vi "Comet Page.vi"() -> ()   [LabVIEW 2017, in "3D Comet.lvclass"]
uses:
  <vilib>/Math Plots/3D Math Plots/3D Comet/3D Comet/3D Comet.lvclass
  <vilib>/Math Plots/3D Math Plots/3D Comet/3D Comet/Typedef/3D Comet Property Array.ctl
  <vilib>/Math Plots/3D Math Plots/3D Comet/3D Comet/Typedef/3D Comet Property.ctl
  <vilib>/Math Plots/3D Math Plots/3D Plot/3D Plot/Typedef/Sprite Type.ctl
  <vilib>/Math Plots/3D Math Plots/3D Plot/3D Plot/Typedef/Line Type.ctl
  <vilib>/Math Plots/3D Math Plots/3D Plot/3D Plot/Typedef/Dialog State.ctl
  <vilib>/Math Plots/3D Math Plots/3D Plot/3D Plot/Typedef/Temp Scene State.ctl
  <vilib>/Math Plots/3D Math Plots/3D Plot/3D Plot/Typedef/Temp Scene Property Action.ctl
  <vilib>/Math Plots/3D Math Plots/3D Plot/3D Plot/3D Plot.lvclass
panel:
  in  "Point Color":u32(colorbox) caption="Point color"
  in  "Point Size":sgl caption="Point size" min=0.001 step=1
  in  "Point Style":u16(ring) caption="Point style"
  in  "Tail Length":sgl caption="Tail length"
  in  "Line Style":u16(ring) caption="Line style"
  in  "Antialiasing":bool
  in  "Line Width":sgl=0.001 caption="Line width" min=0.001 step=1
  in  "Line Color":u32(colorbox) caption="Line color"
  out "Comet Property Out":T1
  in  "Comet Property In":T1
  in  "YZ Plane Projection":bool caption="YZ plane projection"
  in  "XZ Plane Projection":bool caption="XZ plane projection"
  in  "XY plane projection":bool
  in  "Coordinate System":u16(ring) caption="Coordinate system" items=["Cartesian", "Cylindrical", "Spherical"]
  in  "Plot Opacity":sgl(slide) caption="Plot opacity(%)" min=0 max=100 scale=0.0..100.0
  in  "Plot List":i32(listbox)
  in  "Move Down":bool
  in  "Move Up":bool
  in  "Delete":bool
  in  "New":bool
  in  "Event Registration":refnum<event-registration>
  # "Comet"
  # "General"
  # "Projection"
  # "Comet Line"
  # "Comet Point"
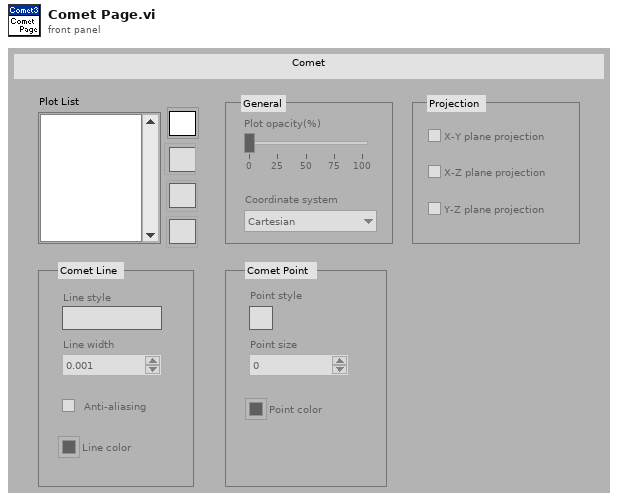
[diagram p1: front panel]
types:
  T1 = typedef "3D Comet.lvclass/3D Comet Property Array.ctl" = T2[]
  T2 = typedef "3D Comet.lvclass/3D Comet Property.ctl" = cluster{"General Property":cluster{"Plot Name":string, "Coordinate System":enum16{"Cartesian", "Cylindrical", "Spherical"}, "Opacity":sgl}, "Projection Property":cluster{"Draw XY":bool, "Draw YZ":bool, "Draw XZ":bool}, "Plot Property":cluster{"Sprite Type":T3, "Point Size":sgl, "Point Color":u32, "Line Style":T4, "Line Width":sgl, "Line Color":u32, "Antialiasing":bool}, "Comet Property":cluster{"Body length":sgl}}
  T3 = typedef "3D Plot.lvclass/Sprite Type.ctl" = enum16{"None", "Empty Square", "Solid Square", "Empty Diamond", "Solid Diamond", "Empty Circle", "Solid Circle", "Asterisk", "Bold X", "Wireframe Sphere", "Solid Sphere", "Wireframe Cube", "Solid Cube"}
  T4 = typedef "3D Plot.lvclass/Line Type.ctl" = enum16{"None", "Solid", "Dash", "Dot", "Dash Dot"}
  T5 = typedef "3D Plot.lvclass/Dialog State.ctl" = enum16{"Initialize", "Read Porperty", "Write Property", "Idle", "Exit"}
  T6 = typedef "3D Plot.lvclass/Temp Scene State.ctl" = enum16{"Create", "Update Scene", "Get Plot Representation", "Destory"}
  T7 = typedef "3D Plot.lvclass/Temp Scene Property Action.ctl" = enum16{"Graph Property", "Light Property", "Axis Property", "Value Pair Property", "Format Property", "Cursor Property", "Plot Specific Property"}
  T8 = typedef "3D Plot.lvclass/Multiplot Representation.ctl" = cluster{"Plot Represention Array":T9[], "Max Range":T10}
  T9 = typedef "3D Plot.lvclass/Plot Representation.ctl" = cluster{"Plot ID":i32, "Plot Range":T10, "Mesh Data":T11, "Dimension":cluster{"X Dimension":i32, "Y Dimension":i32}, "Ramp Range":T10}
  T10 = typedef "3D Plot.lvclass/Range Clusters.ctl" = cluster{"X Range":cluster{"Max X":sgl, "Min X":sgl}, "Y Range":cluster{"Max Y":sgl, "Min Y":sgl}, "Z Range":cluster{"Max Z":sgl, "Min Z":sgl}}
  T11 = typedef "3D Plot.lvclass/Mesh Data.ctl" = cluster{"Index Array":u32[], "Vertex Array":cluster{"X":sgl, "Y":sgl, "Z":sgl}[], "Normal Array":cluster{"X":sgl, "Y":sgl, "Z":sgl}[], "Color Index Array":i32[]}
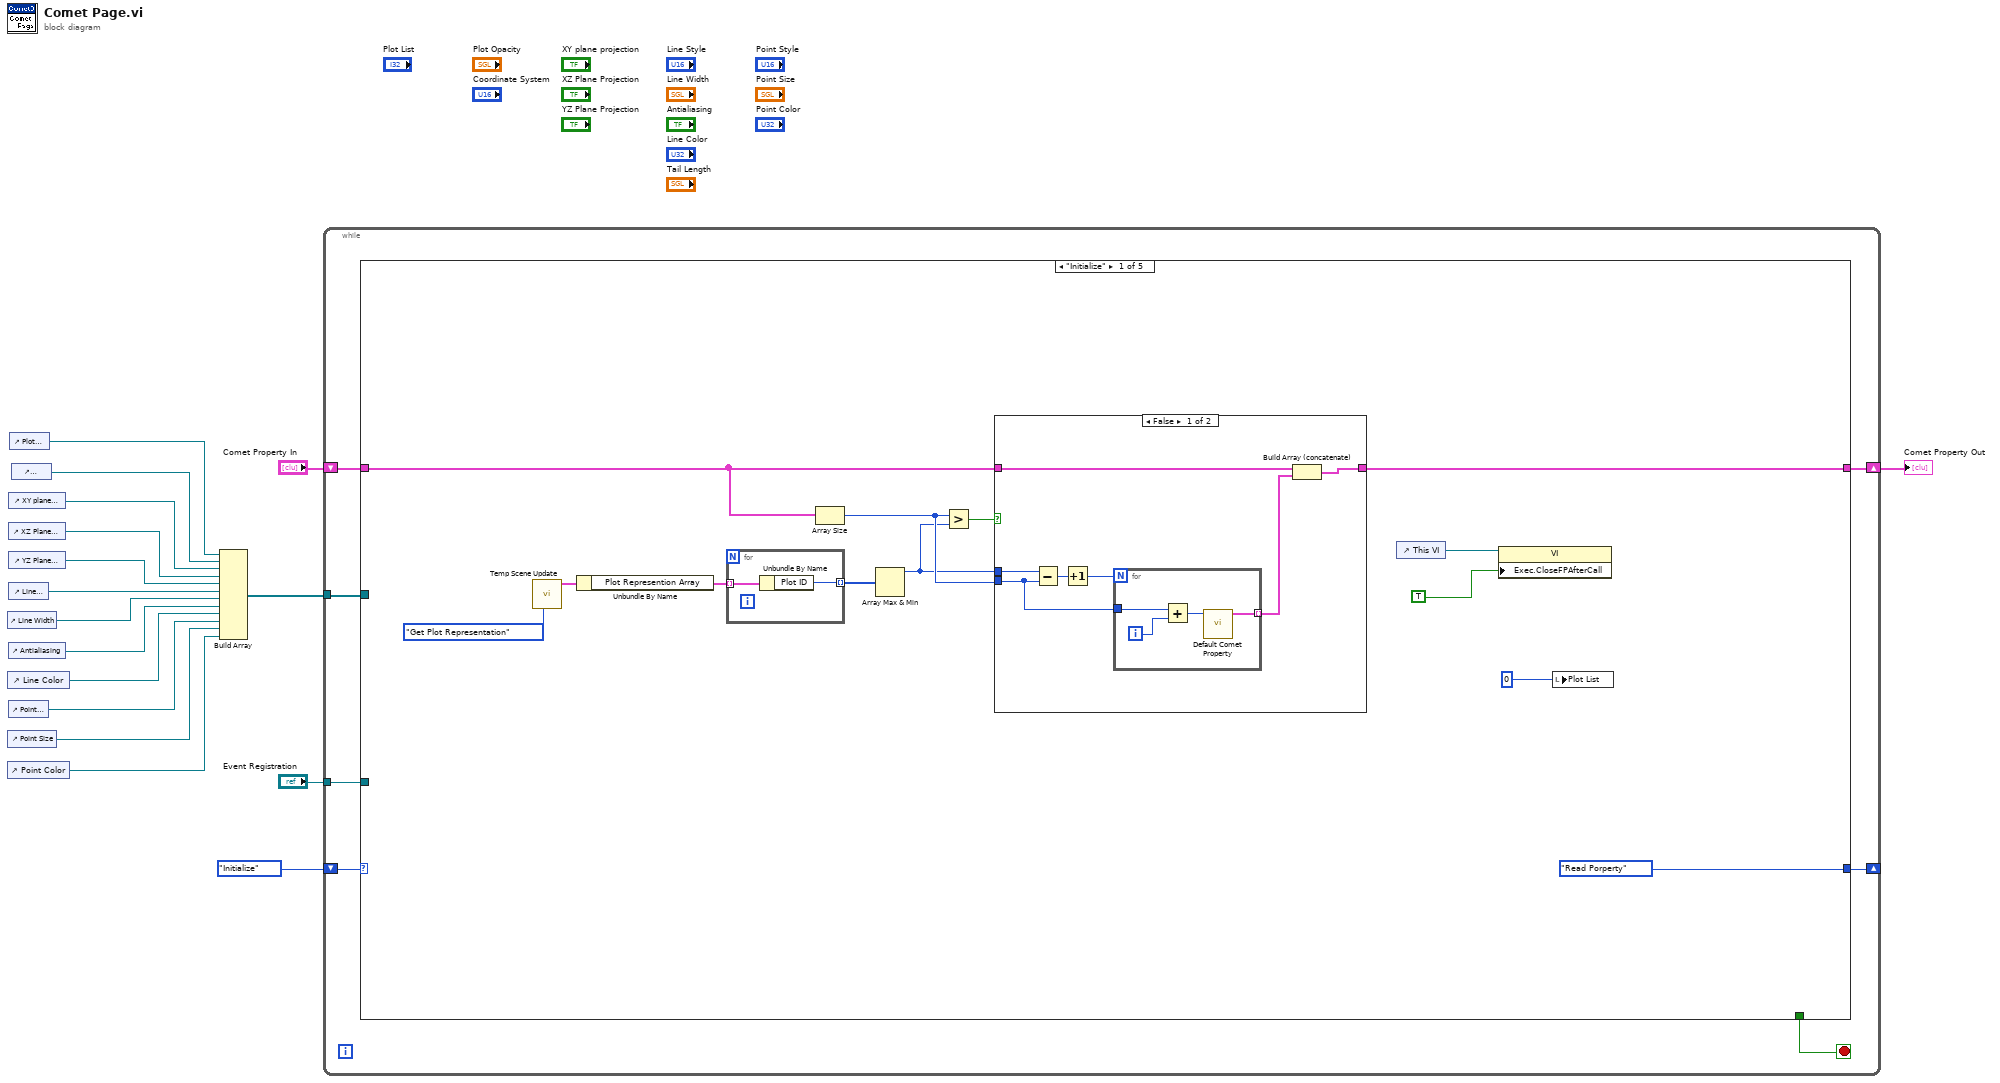
[diagram p0: block diagram]
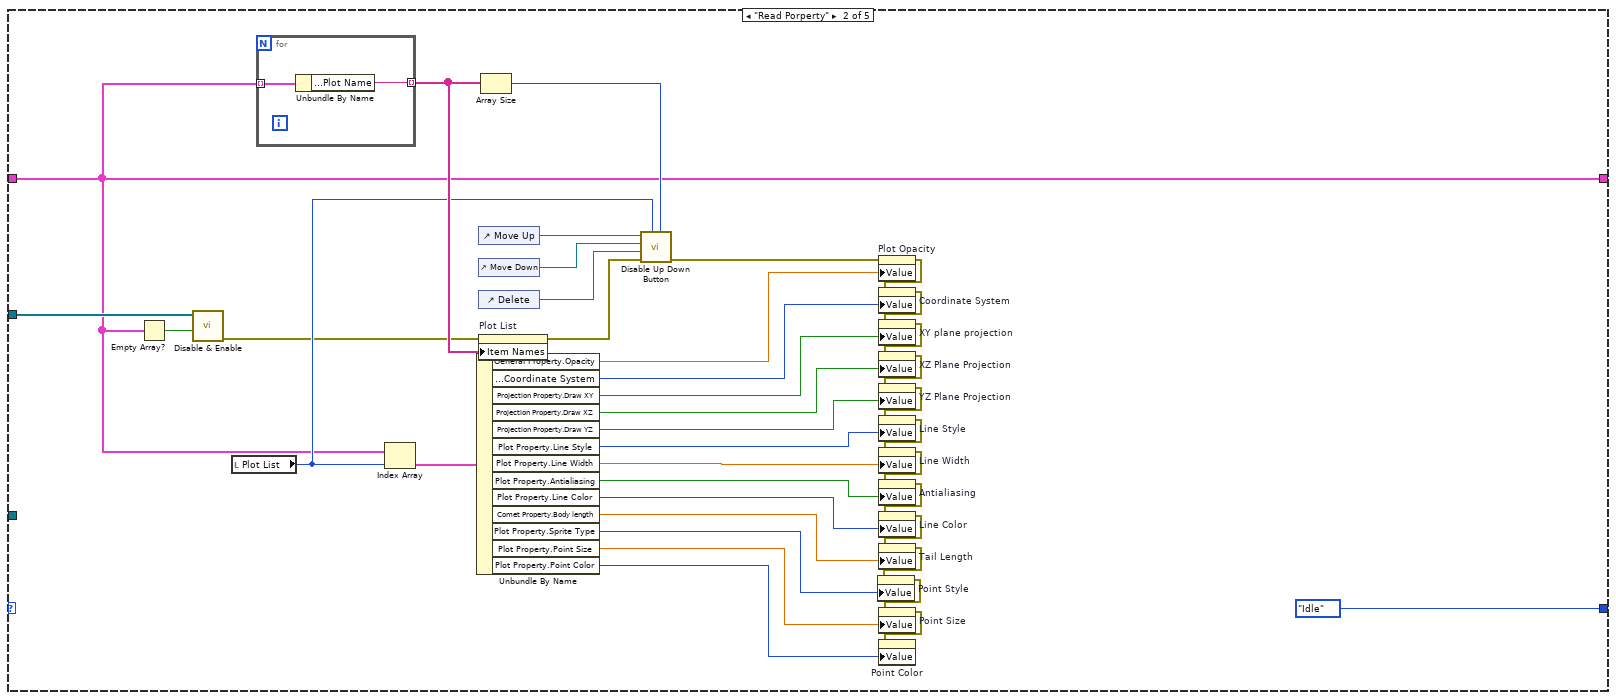
[diagram p3: hidden frame]
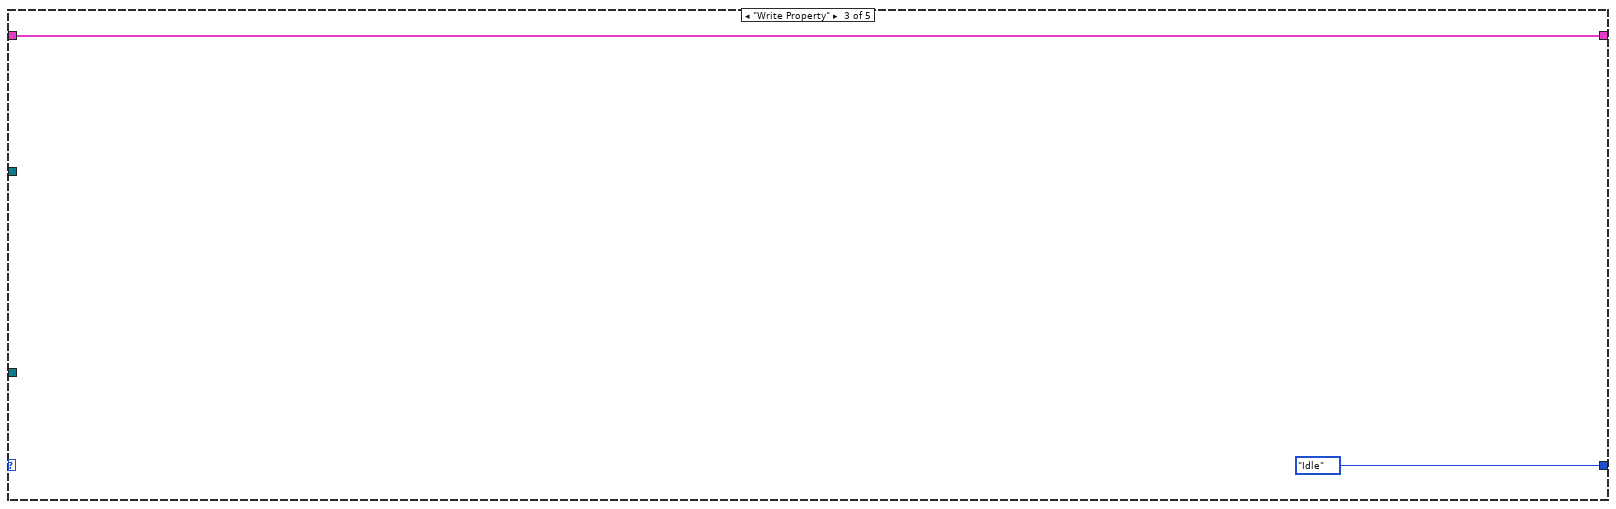
[diagram p4: hidden frame]
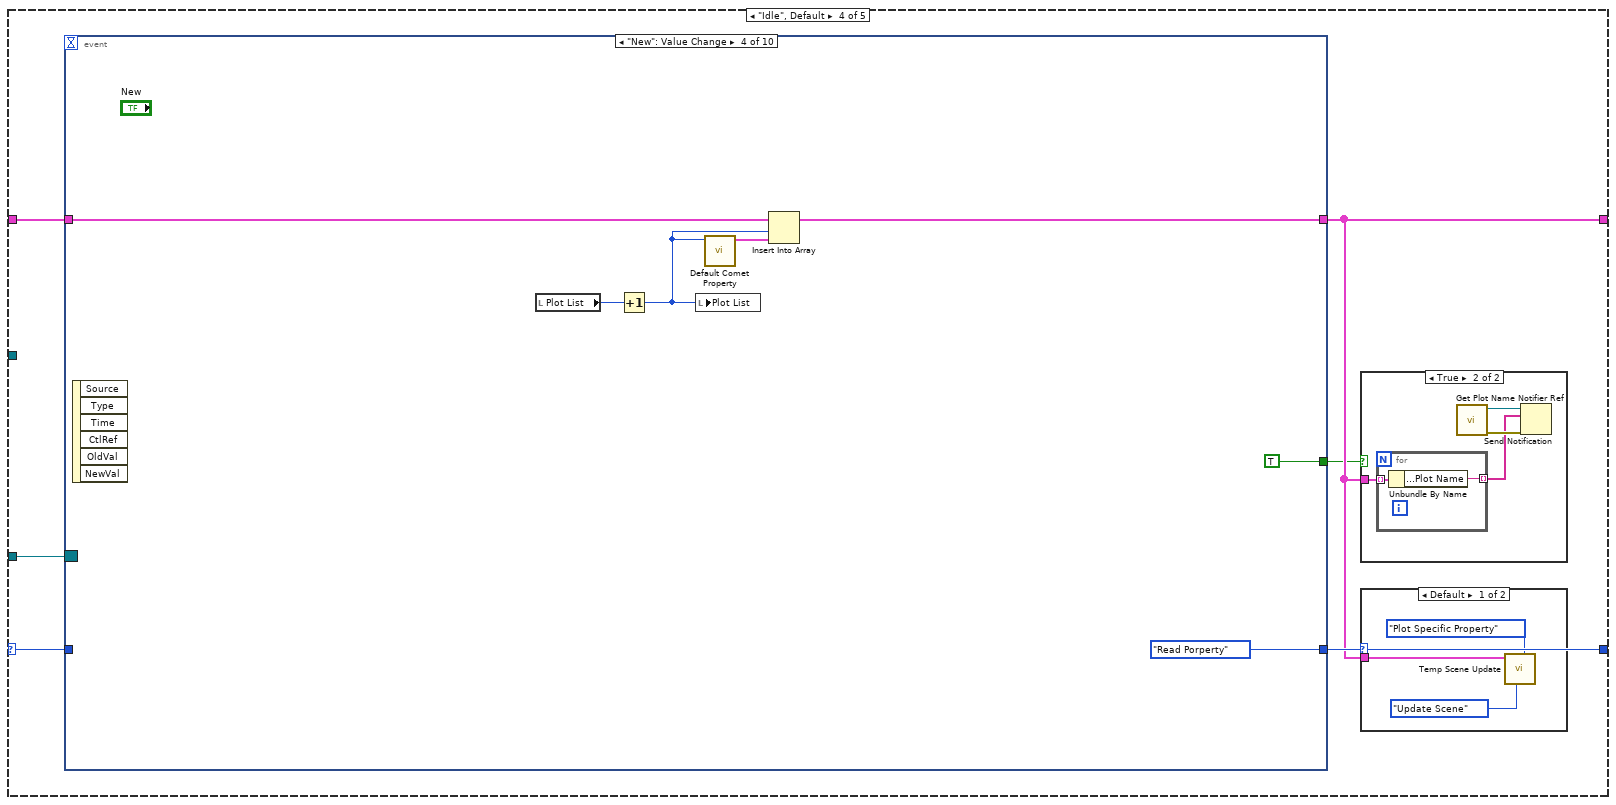
[diagram p5: hidden frame]
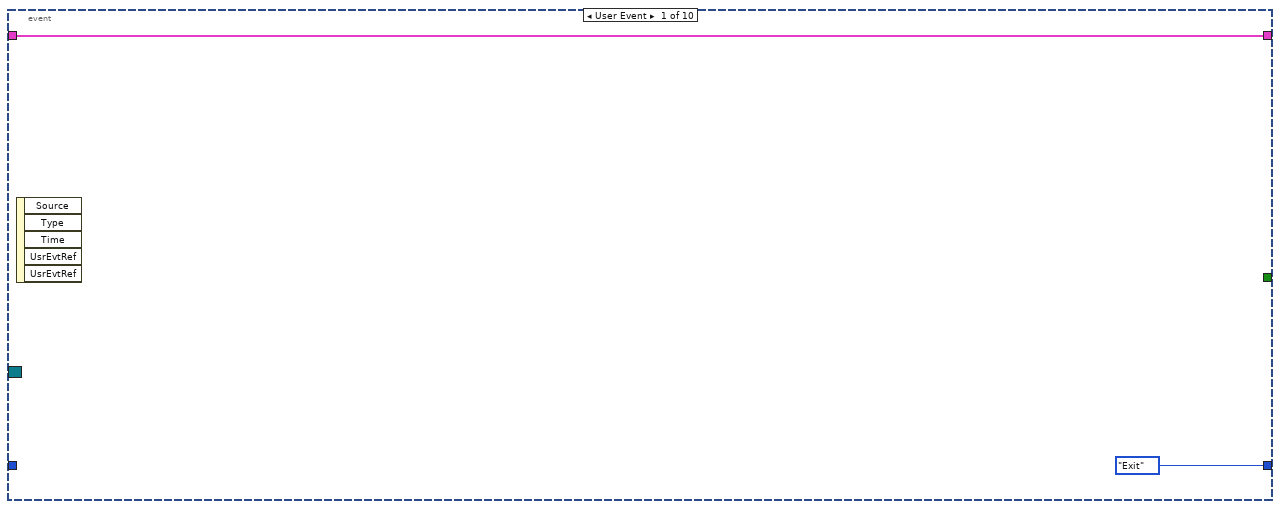
[diagram p8: hidden frame]
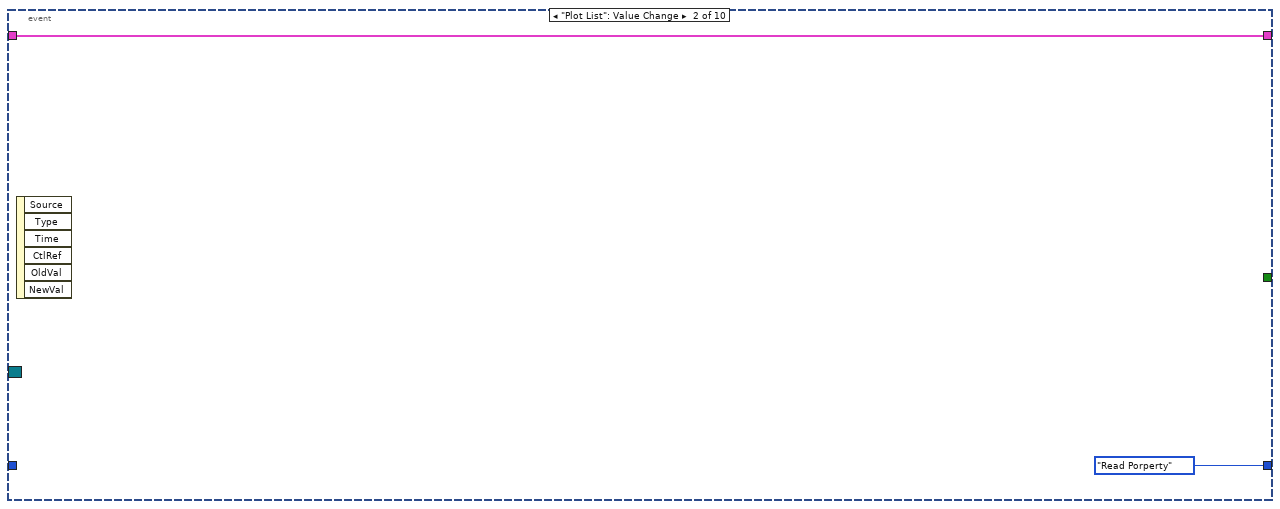
[diagram p9: hidden frame]
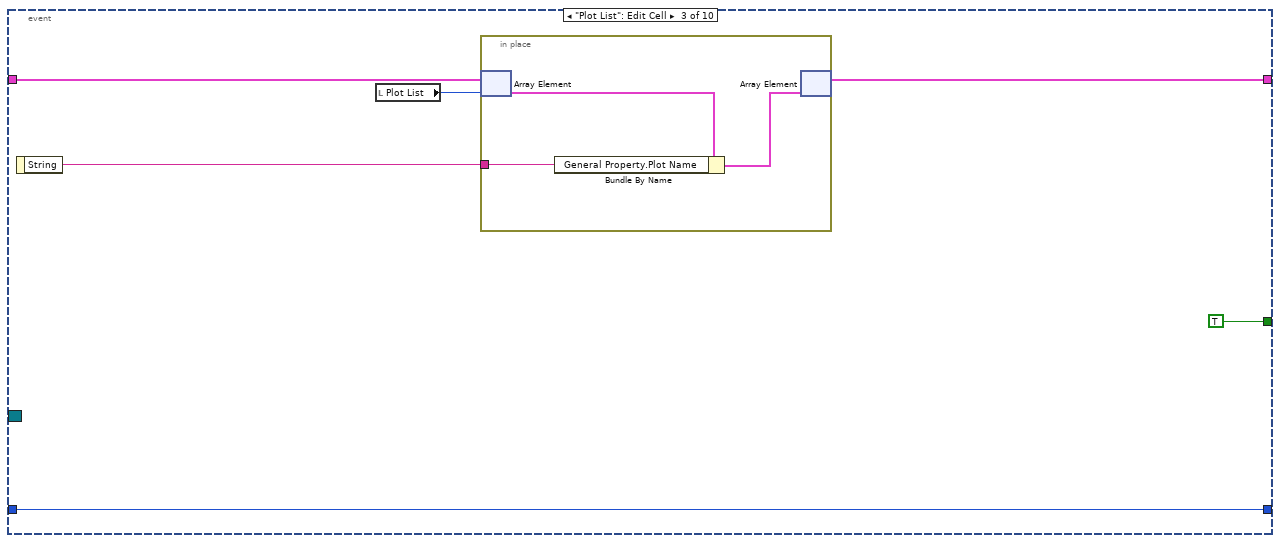
[diagram p10: hidden frame]
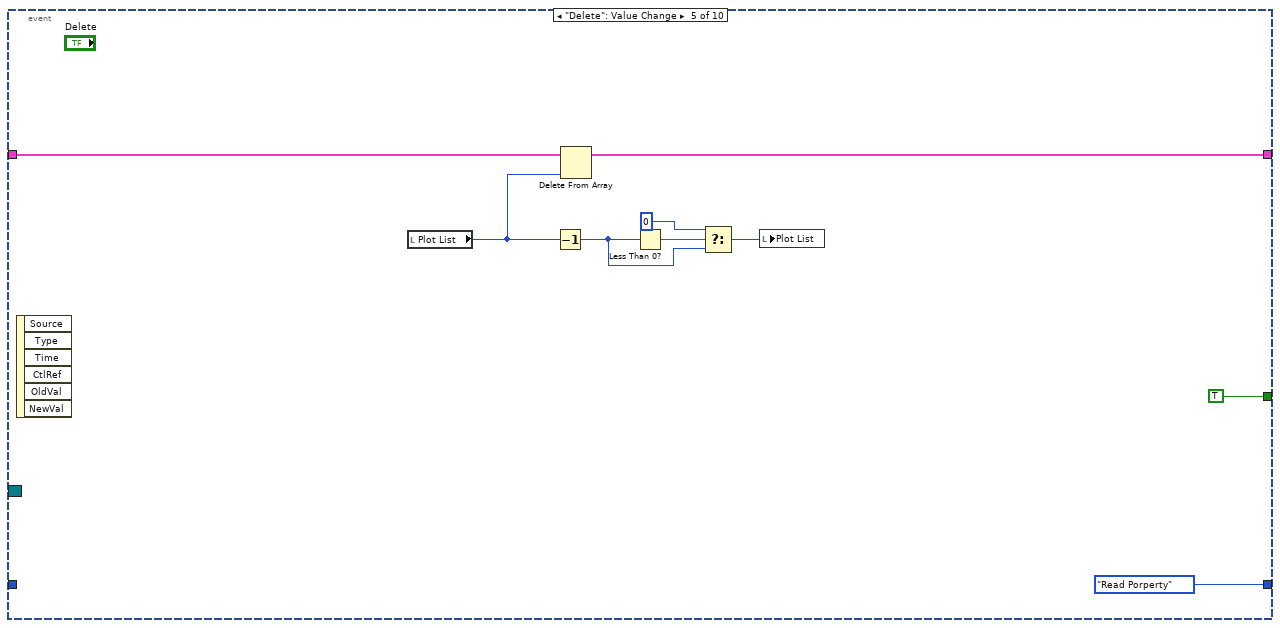
[diagram p11: hidden frame]
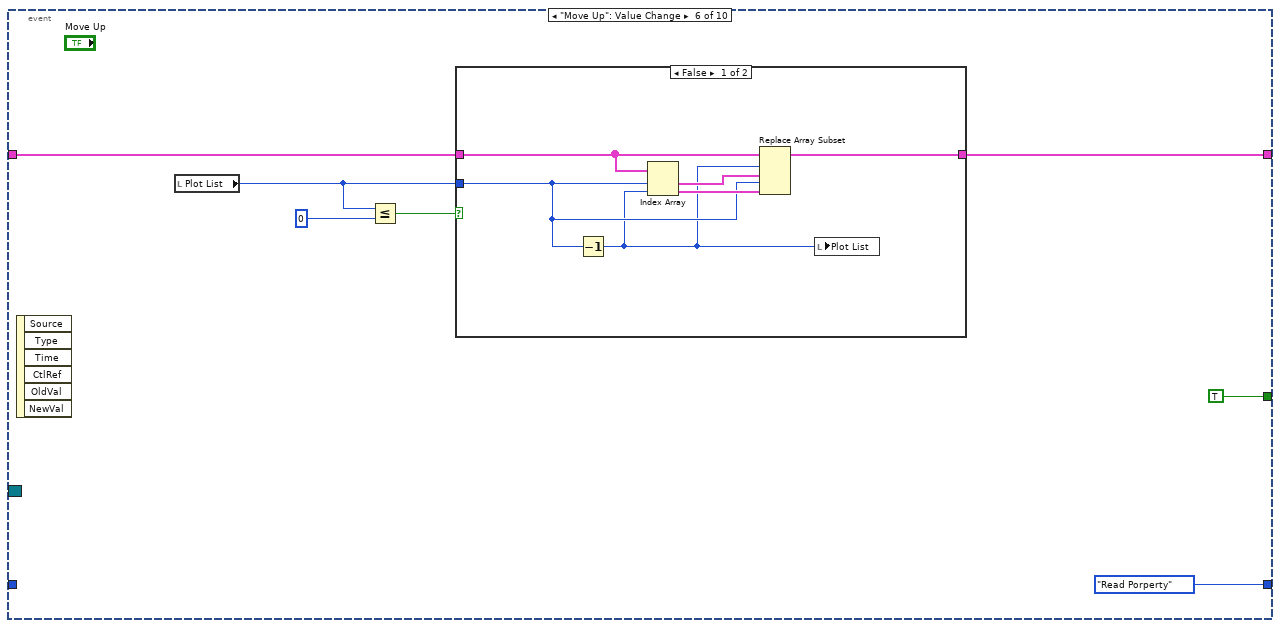
[diagram p12: hidden frame]
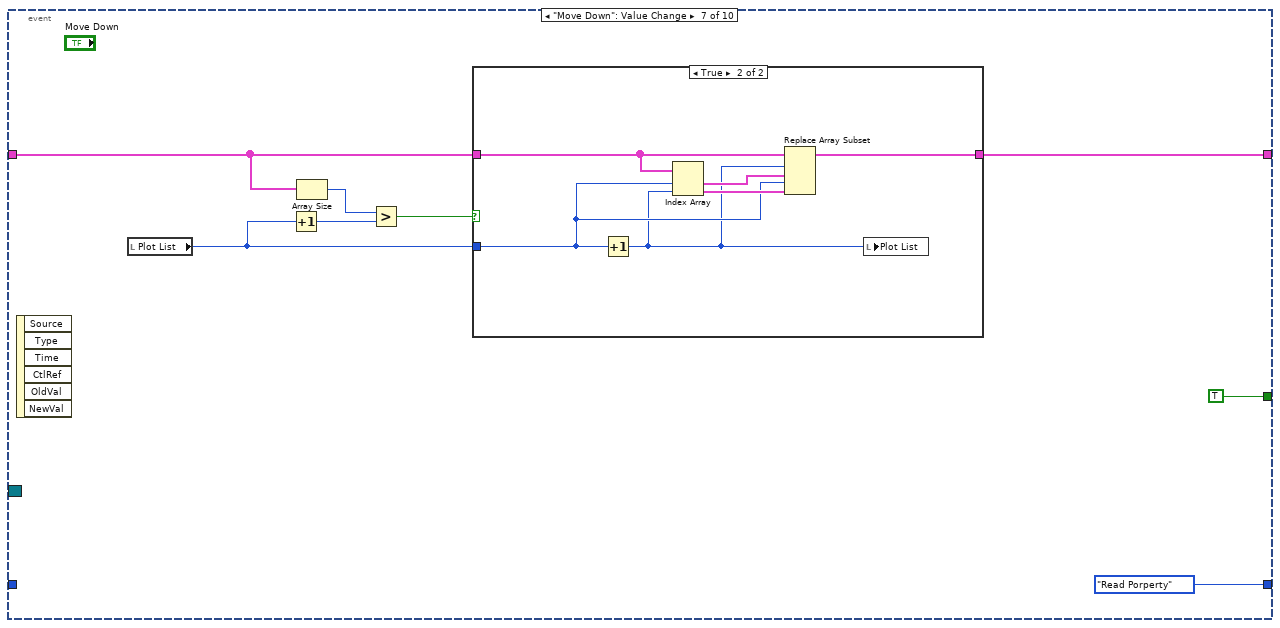
[diagram p14: hidden frame]
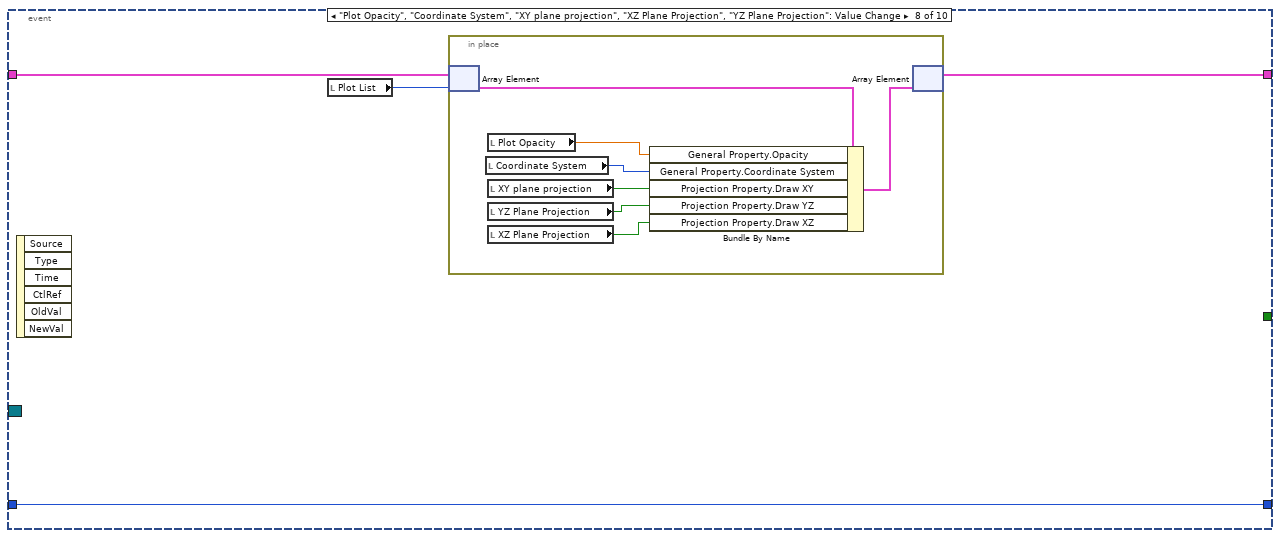
[diagram p16: hidden frame]
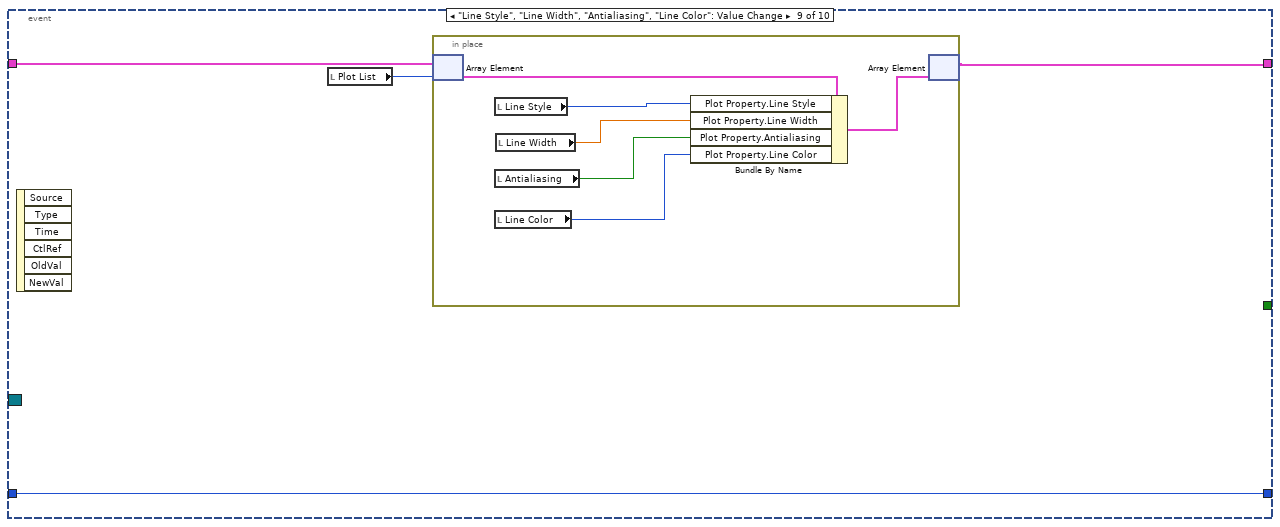
[diagram p17: hidden frame]
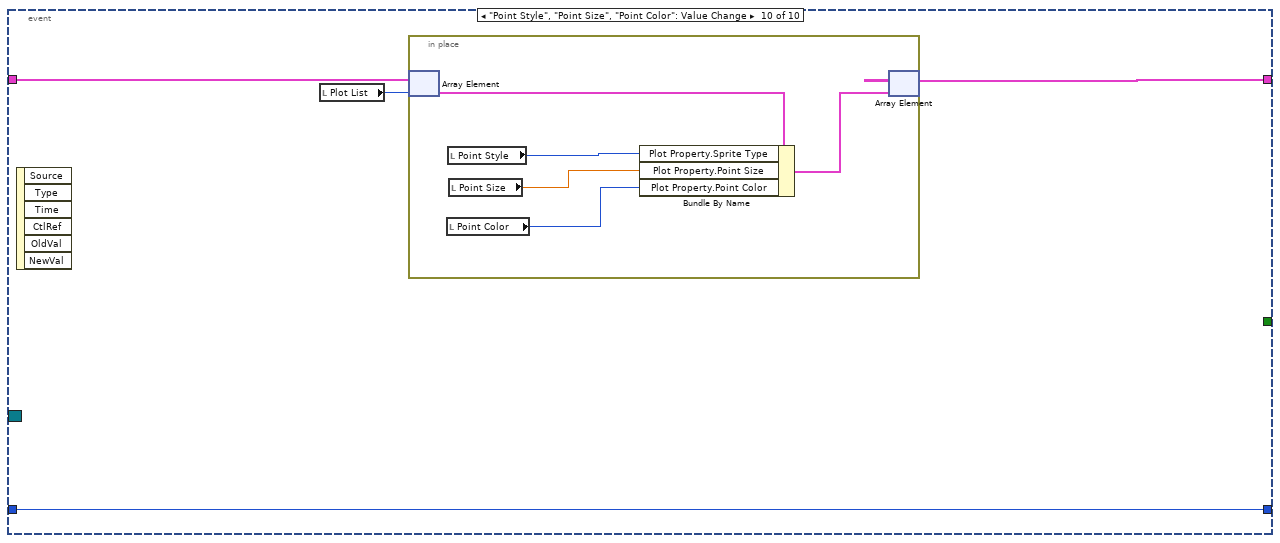
[diagram p18: hidden frame]
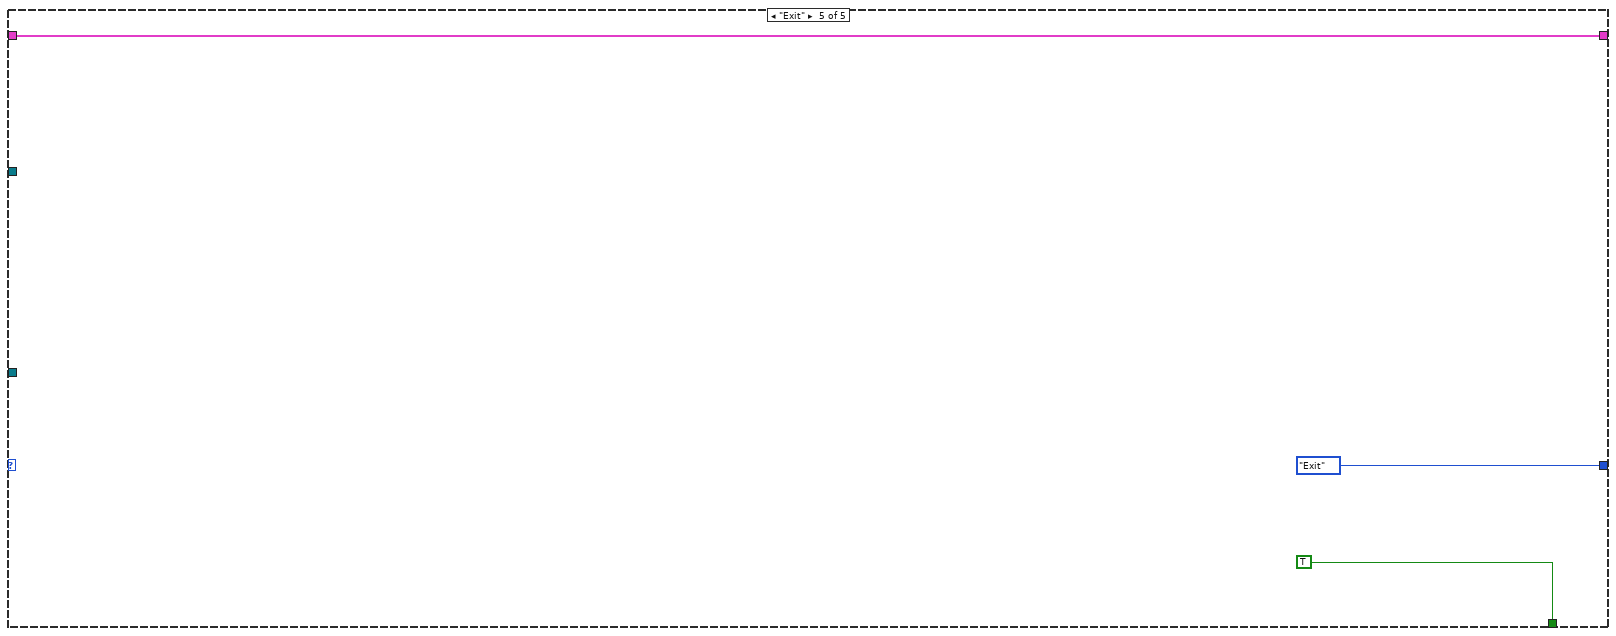
[diagram p19: hidden frame]
diagram:
  n1 = control-ref of="Line Width"() -> (w7:refnum<vi>)
  n2 = control-ref of="Line Color"() -> (w5:refnum<vi>)
  n3 = control-ref of="Point Size"() -> (w3:refnum<vi>)
  n4 = control-ref of="Point Color"() -> (w2:refnum<vi>)
  n5 = control-ref of="XY plane projection"() -> (w11:refnum<vi>)
  n6 = control-ref of="XZ Plane Projection"() -> (w10:refnum<vi>)
  n7 = control-ref of="YZ Plane Projection"() -> (w9:refnum<vi>)
  n8 = control-ref of="Line Style"() -> (w8:refnum<vi>)
  n9 = control-ref of="Antialiasing"() -> (w6:refnum<vi>)
  n10 = control-ref of="Point Style"() -> (w4:refnum<vi>)
  n11 = control-ref of="Plot Opacity"() -> (w13:refnum<vi>)
  n12 = control-ref of="Coordinate System"() -> (w12:refnum<vi>)
  n13 = Build Array(w13, w12, w11, w10, w9, w8, w7, w6, w5, w4, w3, w2) -> (w1:refnum<vi>[])
  n14 = while {
    shift-right: [w23] -> w14
    shift-left: "Comet Property In" -> [w24]
    shift-right: [w19] -> _
    shift-left: Dialog_State."Initialize" -> [w22]
    tunnel: "Event Registration" -> [w20]
    tunnel: w1 -> [w18]
    stop <- w21 stop-if-true
    n15 = case shown="\"Initialize\"" w22 {
      selector: w22 -> [_ _ _ w98 _]
      tunnel: w24 -> [w27 w79 w93 w100 w198]
      tunnel: [w26 w79 w93 w96 w198] -> w23
      tunnel: [Dialog_State."Read Porperty" Dialog_State."Idle" Dialog_State."Idle" w97 Dialog_State."Exit"] -> w19
      tunnel: [_ _ _ _ TRUE] -> w21
      tunnel: w20 -> [_ _ _ w99 _]
      tunnel: w18 -> [_ w80 _ _ _]
      frame "Initialize" {
        n16 = call <vilib>:"Temp Scene Update.vi"("State"=Temp_Scene_State."Get Plot Representation") -> ("Multiplot Representation"=w32:T8)  [unwired: 5 in, 5 out]
        n17 = Unbundle By Name(w32) -> ("Plot Represention Array"=w25:T9[])
        n18 = for {
          tunnel: w25 -> [w51] mode=indexing
          tunnel: [w50] -> w31 mode=indexing
          n19 = Unbundle By Name(w51) -> ("Plot ID"=w50:i32)
        }
        n20 = Array Size(array=w27) -> (size(s)=w29:i32)
        n21 = Array Max & Min(array=w31) -> (max value=w28:i32)  [unwired: 3 out]
        n22 = Greater?(x=w29, y=w28) -> (0:w30:bool)
        n23 = case shown="False" w30 {
          tunnel: [w42 w49] -> w26
          tunnel: w27 -> [w44 w49]
          tunnel: w29 -> [w38 _]
          tunnel: w28 -> [w39 _]
          frame False {
            n24 = Subtract(x=w39, y=w38) -> (x-y=w41:i32)
            n25 = Increment(x=w41) -> (x+1=w40:i32)
            n26 = for {
              N: w40 -> [_]
              tunnel: w38 -> [w47]
              tunnel: [w45] -> w43 mode=indexing
              i -> [w48]
              n27 = Add(x=w47, y=w48) -> (x+y=w46:i32)
              n28 = call <vilib>:"Default Comet Property.vi"("Plot ID"=w46) -> ("Default Property"=w45:T2)  [unwired: 10 out]
            }
            n29 = Build Array (concatenate)(w44, w43) -> (w42:T1)
          }
          frame True {
          }
        }
        n30 = control-ref of="This VI"() -> (w36:refnum<vi>)
        n31 = property class="VI"(reference=w36, "Exec.CloseFPAfterCall"=TRUE ("Execution:Close After Call")) -> ()  [unwired: 1 in, 2 out]
        n32 = local write "Plot List"(0 ("Plot List")) -> ()
      }
      frame "Read Porperty" {
        n33 = Empty Array?(array=w79) -> (empty?=w81:bool)
        n34 = call <vilib>:"Disable & Enable.vi"("Disabled?"=w81, "Control Ref Array"=w80) -> ("error out"=w78:errorcluster)  [unwired: 1 in, 8 out]
        n35 = local read "Plot List"() -> (w82:i32)
        n36 = for {
          tunnel: w79 -> [w92] mode=indexing
          tunnel: [w91] -> w84 mode=indexing
          n37 = Unbundle By Name(w92) -> ("General Property.Plot Name"=w91:string)
        }
        n38 = Index Array(array=w79, index=w82) -> (element=w89:T2)
        n39 = Unbundle By Name(w89) -> ("General Property.Opacity"=w67:sgl, "General Property.Coordinate System"=w66:enum16{"Cartesian", "Cylindrical", "Spherical"}, "Projection Property.Draw XY"=w65:bool, "Projection Property.Draw XZ"=w64:bool, "Projection Property.Draw YZ"=w63:bool, "Plot Property.Line Style"=w62:T4, "Plot Property.Line Width"=w61:sgl, "Plot Property.Antialiasing"=w60:bool, "Plot Property.Line Color"=w59:u32, "Comet Property.Body length"=w58:sgl, "Plot Property.Sprite Type"=w53:T3, "Plot Property.Point Size"=w57:sgl, "Plot Property.Point Color"=w56:u32)
        n40 = control-ref of="Move Up"() -> (w86:refnum<vi>)
        n41 = control-ref of="Move Down"() -> (w87:refnum<vi>)
        n42 = control-ref of="Delete"() -> (w88:refnum<vi>)
        n43 = property on="Plot List" class="LstBox (strict)"(error in=w78, "Item Names"=w84) -> (error out=w83:errorcluster)  [unwired: 1 in, 1 out]
        n44 = Array Size(array=w84) -> (size(s)=w85:i32)
        n45 = call <vilib>:"Disable Up Down Button.vi"("Length"=w85, "Index"=w82, "error in (no error)"=w83, "Delete Ref"=w88, "Move Down Ref"=w87, "Move Up Ref"=w86) -> ("error out"=w52:errorcluster)  [unwired: 5 out]
        n46 = property on="Plot Opacity" class="Slide (strict)"(error in=w52, "Value"=w67) -> (error out=w77:errorcluster)  [unwired: 1 in, 1 out]
        n47 = property on="Coordinate System" class="Ring (strict)"(error in=w77, "Value"=w66) -> (error out=w76:errorcluster)  [unwired: 1 in, 1 out]
        n48 = property on="XY plane projection" class="Bool (strict)"(error in=w76, "Value"=w65) -> (error out=w75:errorcluster)  [unwired: 1 in, 1 out]
        n49 = property on="XZ Plane Projection" class="Bool (strict)"(error in=w75, "Value"=w64) -> (error out=w74:errorcluster)  [unwired: 1 in, 1 out]
        n50 = property on="YZ Plane Projection" class="Bool (strict)"(error in=w74, "Value"=w63) -> (error out=w73:errorcluster)  [unwired: 1 in, 1 out]
        n51 = property on="Line Style" class="Ring (strict)"(error in=w73, "Value"=w62) -> (error out=w72:errorcluster)  [unwired: 1 in, 1 out]
        n52 = property on="Line Width" class="DigNum (strict)"(error in=w72, "Value"=w61) -> (error out=w71:errorcluster)  [unwired: 1 in, 1 out]
        n53 = property on="Antialiasing" class="Bool (strict)"(error in=w71, "Value"=w60) -> (error out=w70:errorcluster)  [unwired: 1 in, 1 out]
        n54 = property on="Line Color" class="ColBox"(error in=w70, "Value"=w59) -> (error out=w69:errorcluster)  [unwired: 1 in, 1 out]
        n55 = property on="Tail Length" class="DigNum (strict)"(error in=w69, "Value"=w58) -> (error out=w55:errorcluster)  [unwired: 1 in, 1 out]
        n56 = property on="Point Style" class="Ring (strict)"(error in=w55, "Value"=w53) -> (error out=w54:errorcluster)  [unwired: 1 in, 1 out]
        n57 = property on="Point Size" class="DigNum (strict)"(error in=w54, "Value"=w57) -> (error out=w68:errorcluster)  [unwired: 1 in, 1 out]
        n58 = property on="Point Color" class="ColBox"(error in=w68, "Value"=w56) -> ()  [unwired: 1 in, 2 out]
      }
      frame "Write Property" {
      }
      frame "Idle", Default {
        n59 = event shown="[3] \"New\": Value Change" {
          selector: w99 -> [_ _ _ _ _ _ _ _ _ _]
          dyn-events: _ -> [_ _ _ _ _ _ _ _ _ _]
          timeout: _ -> [_ _ _ _ _ _ _ _ _ _]
          tunnel: w100 -> [w111 w113 w117 w127 w136 w141 w155 w169 w180 w190]
          tunnel: [w111 w113 w116 w126 w137 w140 w154 w168 w179 w189] -> w96
          tunnel: [Dialog_State."Exit" Dialog_State."Read Porperty" w115 Dialog_State."Read Porperty" Dialog_State."Read Porperty" Dialog_State."Read Porperty" Dialog_State."Read Porperty" w171 w182 w191] -> w97
          tunnel: w98 -> [_ _ w115 _ _ _ _ w171 w182 w191]
          tunnel: [_ _ TRUE TRUE TRUE TRUE TRUE _ _ _] -> w95
          event User Event {
            n60 = event-data() -> ()  [unwired: 6 out]
          }
          event "Plot List": Value Change {
            n61 = event-data() -> ()  [unwired: 7 out]
          }
          event "Plot List": Edit Cell {
            n62 = event-data() -> ("String"=w118:string)  [unwired: 1 out]
            n63 = local read "Plot List"() -> (w119:i32)
            n64 = in-place {
              in-place-border: w118 -> [w120]
              n65 = in-place-array #1(w117, w119) -> (w122:T2)
              n66 = Bundle By Name(cluster=w122, "General Property.Plot Name"=w120) -> (w121:T2)
              n67 = in-place-array #1(w121) -> (w116:T1)  [unwired: 1 out]
            }
          }
          event "New": Value Change {
            n68 = event-data() -> ()  [unwired: 7 out]
            n69 = local read "Plot List"() -> (w128:i32)
            n70 = Increment(x=w128) -> (x+1=w124:i32)
            n71 = local write "Plot List"(w124) -> ()
            n72 = call <vilib>:"Default Comet Property.vi"("Plot ID"=w124) -> ("Default Property"=w123:T2)  [unwired: 10 out]
            n73 = Insert Into Array(array=w127, index=w124, new element=w123) -> (w126:T1)
          }
          event "Delete": Value Change {
            n74 = event-data() -> ()  [unwired: 7 out]
            n75 = local read "Plot List"() -> (w132:i32)
            n76 = Decrement(x=w132) -> (x-1=w133:i32)
            n77 = Delete From Array(array=w136, index=w132) -> (array with subset deleted=w137:T1)  [unwired: 1 in, 1 out]
            n78 = Less Than 0?(x=w133) -> (x < 0?=w135:bool)
            n79 = Select(t=0, s=w135, f=w133) -> (s? t:f=w131:i32)
            n80 = local write "Plot List"(w131) -> ()
          }
          event "Move Up": Value Change {
            n81 = event-data() -> ()  [unwired: 7 out]
            n82 = local read "Plot List"() -> (w142:i32)
            n83 = Less Or Equal?(x=w142, y=0) -> (x <= y?=w143:bool)
            n84 = case shown="False" w143 {
              tunnel: w141 -> [w149 w152]
              tunnel: [w148 w152] -> w140
              tunnel: w142 -> [w147 _]
              frame False {
                n85 = Decrement(x=w147) -> (x-1=w146:i32)
                n86 = Index Array(array=w149, index #1=w147, index #2=w146) -> (element #1=w151:T2, element #2=w150:T2)
                n87 = Replace Array Subset(array=w149, new element #1=w151, index #1=w146, new element #2=w150, index #2=w147) -> (w148:T1)
                n88 = local write "Plot List"(w146) -> ()
              }
              frame True {
                # "List value is less or equal to 0.\nThe active item is in the top of the list."
              }
            }
          }
          event "Move Down": Value Change {
            n89 = event-data() -> ()  [unwired: 7 out]
            n90 = local read "Plot List"() -> (w156:i32)
            n91 = Increment(x=w156) -> (x+1=w158:i32)
            n92 = Array Size(array=w155) -> (size(s)=w159:i32)
            n93 = Greater?(x=w159, y=w158) -> (0:w157:bool)
            n94 = case shown="True" w157 {
              tunnel: w155 -> [w161 w165]
              tunnel: [w161 w164] -> w154
              tunnel: w156 -> [_ w163]
              frame False {
                # "List value +1 is not less array length.\nThe active item is in the buttom of the list."
              }
              frame True {
                n95 = Increment(x=w163) -> (x+1=w162:i32)
                n96 = Index Array(array=w165, index #1=w163, index #2=w162) -> (element #1=w167:T2, element #2=w166:T2)
                n97 = Replace Array Subset(array=w165, new element #1=w167, index #1=w162, new element #2=w166, index #2=w163) -> (w164:T1)
                n98 = local write "Plot List"(w162) -> ()
              }
            }
          }
          event "Plot Opacity", "Coordinate System", "XY plane projection", "XZ Plane Projection", "YZ Plane Projection": Value Change {
            n99 = event-data() -> ()  [unwired: 7 out]
            n100 = local read "Plot List"() -> (w170:i32)
            n101 = in-place {
              n102 = in-place-array #2(w169, w170) -> (w174:T2)
              n103 = local read "Coordinate System"() -> (w172:u16)
              n104 = local read "Plot Opacity"() -> (w178:sgl)
              n105 = local read "XY plane projection"() -> (w177:bool)
              n106 = local read "YZ Plane Projection"() -> (w175:bool)
              n107 = local read "XZ Plane Projection"() -> (w176:bool)
              n108 = Bundle By Name(cluster=w174, "General Property.Opacity"=w178, "General Property.Coordinate System"=w172, "Projection Property.Draw XY"=w177, "Projection Property.Draw YZ"=w175, "Projection Property.Draw XZ"=w176) -> (w173:T2)
              n109 = in-place-array #2(w173) -> (w168:T1)  [unwired: 1 out]
            }
          }
          event "Line Style", "Line Width", "Antialiasing", "Line Color": Value Change {
            n110 = event-data() -> ()  [unwired: 7 out]
            n111 = local read "Plot List"() -> (w181:i32)
            n112 = in-place {
              n113 = in-place-array #3(w180, w181) -> (w185:T2)
              n114 = local read "Line Style"() -> (w188:u16)
              n115 = local read "Antialiasing"() -> (w186:bool)
              n116 = local read "Line Color"() -> (w183:u32)
              n117 = local read "Line Width"() -> (w187:sgl)
              n118 = Bundle By Name(cluster=w185, "Plot Property.Line Style"=w188, "Plot Property.Line Width"=w187, "Plot Property.Antialiasing"=w186, "Plot Property.Line Color"=w183) -> (w184:T2)
              n119 = in-place-array #3(w184) -> (w179:T1)  [unwired: 1 out]
            }
          }
          event "Point Style", "Point Size", "Point Color": Value Change {
            n120 = event-data() -> ()  [unwired: 7 out]
            n121 = local read "Plot List"() -> (w192:i32)
            n122 = in-place {
              n123 = in-place-array #4(w190, w192) -> (w197:T2)
              n124 = local read "Point Color"() -> (w193:u32)
              n125 = local read "Point Style"() -> (w194:u16)
              n126 = local read "Point Size"() -> (w195:sgl)
              n127 = Bundle By Name(cluster=w197, "Plot Property.Sprite Type"=w194, "Plot Property.Point Size"=w195, "Plot Property.Point Color"=w193) -> (w196:T2)
              n128 = in-place-array #4(w196) -> (w189:T1)  [unwired: 1 out]
            }
          }
        }
        n129 = case shown="True" w95 {
          tunnel: w96 -> [_ w101]
          frame False {
          }
          frame True {
            n130 = for {
              tunnel: w101 -> [w106] mode=indexing
              tunnel: [w105] -> w102 mode=indexing
              n131 = Unbundle By Name(w106) -> ("General Property.Plot Name"=w105:string)
            }
            n132 = call <vilib>:"Get Plot Name Notifier Ref.vi"() -> ("error out"=w104:errorcluster, "Plot Names Notifier Ref"=w103:refnum<notifier>)  [unwired: 1 in, 9 out]
            n133 = Send Notification(notification=w102, notifier=w103, error in (no error)=w104) -> ()  [unwired: 2 out]
          }
        }
        n134 = case shown="Default" w97 {
          tunnel: w96 -> [w109 _]
          frame Default {
            n135 = call <vilib>:"Temp Scene Update.vi"("Property Name"=Temp_Scene_Property_Action."Plot Specific Property", "State"=Temp_Scene_State."Update Scene", "Property In"=w109) -> ()  [unwired: 3 in, 6 out]
          }
          frame "Exit" {
          }
        }
      }
      frame "Exit" {
      }
    }
  }
  "Comet Property Out" <- w14
